vi "RPC Method NIMeasurementServices_RegistryService_RegisterService.vi"(8 "error in (no error)":errorcluster, 10 "Request Data":T2, 11 "gRPC Client in":refnum<class "Discovery_client.lvclass">) -> (0 "error out":errorcluster, 2 "Response Data":T1, 3 "gRPC Client out":refnum<class "Discovery_client.lvclass">)   [LabVIEW 2019, in "Discovery_client.lvlib" / "Discovery_client.lvclass"]
uses:
  Discovery_client.lvclass
  RPC Messages/NIMeasurementServices_RegisterServiceRequest/NIMeasurementServices_RegisterServiceRequest_Data.ctl
  RPC Messages/NIMeasurementServices_ServiceDescriptor/NIMeasurementServices_ServiceDescriptor_Data.ctl
  RPC Messages/NIMeasurementServices_ServiceLocation/NIMeasurementServices_ServiceLocation_Data.ctl
  RPC Messages/NIMeasurementServices_RegisterServiceResponse/NIMeasurementServices_RegisterServiceResponse_Data.ctl
  Discovery_client.lvclass/Discovery_client.ctl
  fa22ca14-33b2-4bc3-8699-3f27c9b27c9c.vi
  <vilib>/gRPC/LabVIEW gRPC Library/Server API/Server/Get Server DLL Path.vi
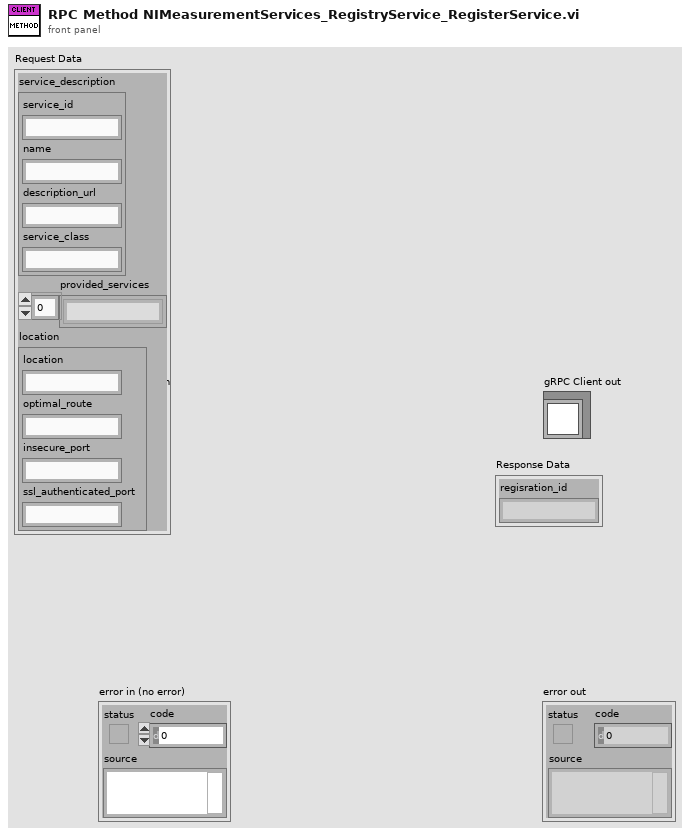
[diagram p1: front panel]
types:
  T1 = typedef "Discovery_client.lvlib/Discovery_client.lvclass/NIMeasurementServices_RegisterServiceResponse_Data.ctl" = cluster{"regisration_id":string}
  T2 = typedef "Discovery_client.lvlib/Discovery_client.lvclass/NIMeasurementServices_RegisterServiceRequest_Data.ctl" = cluster{"service_description":T3, "provided_services":string[], "location":T4}
  T3 = typedef "Discovery_client.lvlib/Discovery_client.lvclass/NIMeasurementServices_ServiceDescriptor_Data.ctl" = cluster{"service_id":string, "name":string, "description_url":string, "service_class":string}
  T4 = typedef "Discovery_client.lvlib/Discovery_client.lvclass/NIMeasurementServices_ServiceLocation_Data.ctl" = cluster{"location":string, "optimal_route":string, "insecure_port":string, "ssl_authenticated_port":string}
  T5 = typedef "gprc-lvsupport-release.lvlib/grpcId.ctl" = u64
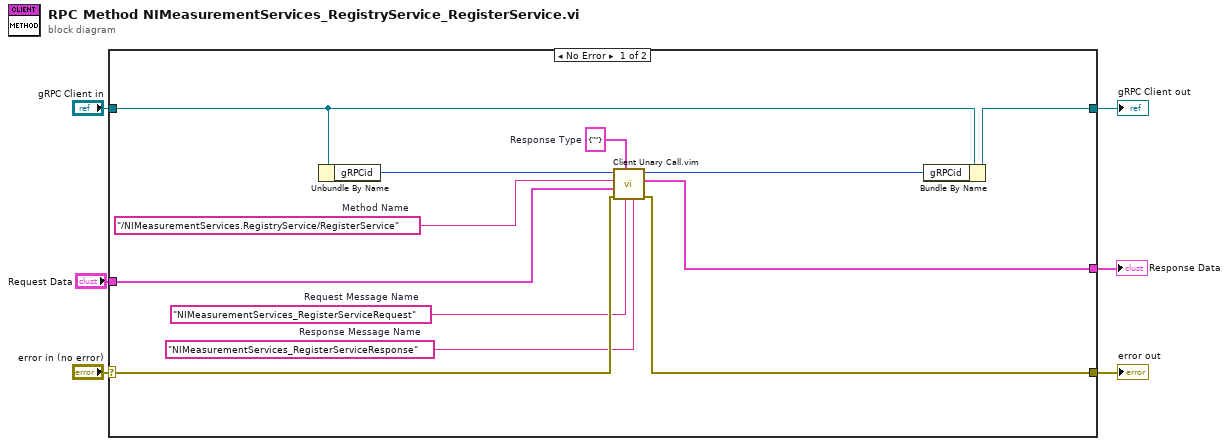
[diagram p0: block diagram]
diagram:
  n1 = case shown="No Error" "error in (no error)" {
    selector: "error in (no error)" -> [w14 w20]
    tunnel: [w13 w20] -> w5
    tunnel: [w15 w19] -> w3
    tunnel: "gRPC Client in" -> [w17 w19]
    tunnel: "Request Data" -> [w11 _]
    tunnel: [w10 _] -> w1
    frame No Error {
      w7 = "NIMeasurementServices_RegisterServiceResponse"  # Response Message Name
      w8 = "NIMeasurementServices_RegisterServiceRequest"  # Request Message Name
      w9 = T1 {"regisration_id"=""}  # Response Type
      w12 = "/NIMeasurementServices.RegistryService/RegisterService"  # Method Name
      n2 = Unbundle By Name(w17) -> ("gRPCid"=w18:T5)
      n3 = call "Client Unary Call.vim"("Response Message Name"=w7, "Request Message Name"=w8, "Response Type"=w9, "error in (no error)"=w14, "Request Data"=w11, "Method Name"=w12, "Client Ref"=w18) -> ("error out"=w13:errorcluster, "Response Data"=w10:T1, "Client Ref Out"=w16:u64)  [unwired: 2 in]
      n4 = Bundle By Name(cluster=w17, "gRPCid"=w16) -> (w15:refnum<class "Discovery_client.lvclass">)
    }
    frame Error {
    }
  }
  "error out" <- w5
  "gRPC Client out" <- w3
  "Response Data" <- w1
